vi "Set Object Size.vi"(4 "Set Width?":bool=TRUE, 6 "Set Height?":bool=TRUE, 7 "Cluster Border Correction":i32, 8 "error in (no error)":errorcluster, 9 "Size":cluster{"width":i16, "height":i16}, 10 "Size":i16, 11 "GObj Refnum":refnum<vi>) -> (0 "error out":errorcluster)   [LabVIEW 2021, in "IObject.lvclass"]
uses:
  IObject.lvclass
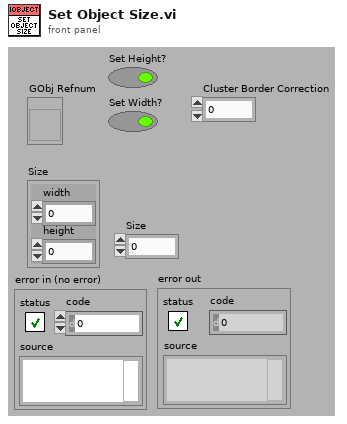
[diagram p1: front panel]
types:
  T1 = typedef "LVBoundsTypeDef.ctl" = cluster{"Width":u32, "Height":u32}
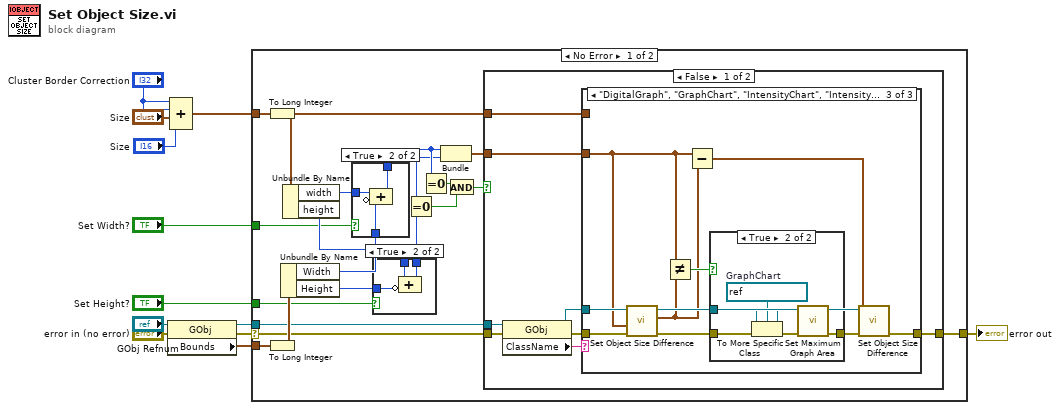
[diagram p0: block diagram]
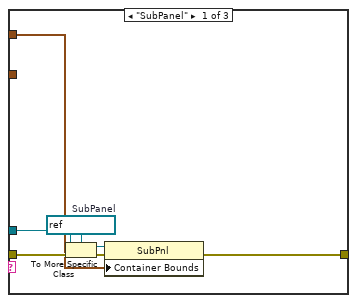
[diagram p2: hidden frame]
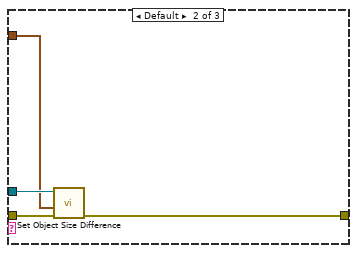
[diagram p3: hidden frame]
diagram:
  n1 = property class="GObj"(reference="GObj Refnum", error in="error in (no error)") -> (reference out=w1:refnum<vi>, error out=w2:errorcluster, "Bounds"=w10:T1)
  n2 = Compound Arithmetic op=unknown("Cluster Border Correction", "Cluster Border Correction", "Size", "Size") -> (w7:cluster{"width":i32, "height":i32})
  n3 = case shown="No Error" w2 {
    selector: w2 -> [w19 w74]
    tunnel: w7 -> [w17 _]
    tunnel: [w26 w74] -> w12
    tunnel: w10 -> [w30 _]
    tunnel: "Set Width?" -> [w22 _]
    tunnel: "Set Height?" -> [w21 _]
    tunnel: w1 -> [w18 _]
    frame No Error {
      n4 = To Long Integer(number=w17) -> (32bit integer=w16:cluster{"width":i32, "height":i32})
      n5 = To Long Integer(number=w30) -> (32bit integer=w31:cluster{"Width":i32, "Height":i32})
      n6 = Unbundle By Name(w31) -> ("Width"=w29:i32, "Height"=w25:i32)
      n7 = Unbundle By Name(w16) -> ("width"=w28:i32, "height"=w27:i32)
      n8 = case shown="True" w22 {
        tunnel: [_ w70] -> w15
        tunnel: w29 -> [_ w69]
        tunnel: w28 -> [_ w68]
        frame False {
        }
        frame True {
          n9 = Compound Arithmetic op=ADD(w68, invert w69) -> (w70:i32)
        }
      }
      n10 = case shown="True" w21 {
        tunnel: [_ w73] -> w14
        tunnel: w27 -> [_ w72]
        tunnel: w25 -> [_ w71]
        frame False {
        }
        frame True {
          n11 = Compound Arithmetic op=ADD(w72, invert w71) -> (w73:i32)
        }
      }
      n12 = Equal To 0?(x=w14) -> (x = 0?=w23:bool)
      n13 = Equal To 0?(x=w15) -> (x = 0?=w24:bool)
      n14 = Bundle(w15, w14) -> (w13:cluster{i32, i32})  [unwired: 1 in]
      n15 = And(x=w24, y=w23) -> (x .and. y?=w20:bool)
      n16 = case shown="False" w20 {
        tunnel: [w39 w67] -> w26
        tunnel: w19 -> [w38 w67]
        tunnel: w18 -> [w36 _]
        tunnel: w16 -> [w33 _]
        tunnel: w13 -> [w32 _]
        frame False {
          n17 = property class="GObj"(reference=w36, error in=w38) -> (reference out=w34:refnum<vi>, error out=w37:errorcluster, "ClassName"=w35:string)
          n18 = case shown="\"DigitalGraph\", \"GraphChart\", \"IntensityChart\", \"IntensityGraph\", \"MixedSignalGraph\", \"WaveformChart\", \"WaveformGraph\", \"XYGraph\"" w35 {
            tunnel: [w45 w48 w56] -> w39
            tunnel: w37 -> [w46 w49 w59]
            tunnel: w34 -> [w44 w50 w54]
            tunnel: w33 -> [w40 _ _]
            tunnel: w32 -> [_ w47 w53]
            frame "SubPanel" {
              w43 = refnum<vi> refnum  # SubPanel
              n19 = To More Specific Class(target class=w43, reference=w44, error in=w46) -> (specific class reference=w41:refnum<vi>, error out=w42:errorcluster)
              n20 = property class="SubPnl"(reference=w41, error in=w42, "Container Bounds"=w40) -> (error out=w45:errorcluster)  [unwired: 1 out]
            }
            frame Default {
              n21 = call "Set Object Size Difference.vi"("error in (no error)"=w49, "dSize"=w47, "GObj Refnum"=w50) -> ("error out"=w48:errorcluster)  [unwired: 7 in, 1 out]
            }
            frame "DigitalGraph", "GraphChart", "IntensityChart", "IntensityGraph", "MixedSignalGraph", "WaveformChart", "WaveformGraph", "XYGraph" {
              n22 = call "Set Object Size Difference.vi"("error in (no error)"=w59, "dSize"=w53, "GObj Refnum"=w54) -> ("error out"=w58:errorcluster, "dSize"=w52:cluster{"width":i32, "height":i32})  [unwired: 7 in]
              n23 = Not Equal?(x=w53, y=w52) -> (x != y?=w57:bool)
              n24 = Subtract(x=w53, y=w52) -> (x-y=w51:cluster{i32, i32})
              n25 = case shown="True" w57 {
                tunnel: [w60 w66] -> w55
                tunnel: w54 -> [_ w65]
                tunnel: w58 -> [w60 w63]
                frame False {
                }
                frame True {
                  w61 = refnum<vi> refnum  # GraphChart
                  n26 = To More Specific Class(target class=w61, reference=w65, error in=w63) -> (specific class reference=w64:refnum<vi>, error out=w62:errorcluster)
                  n27 = call "Set Maximum Graph Area.vi"("error in (no error)"=w62, "Waveform Chart"=w64) -> ("error out"=w66:errorcluster)  [unwired: 9 in]
                }
              }
              n28 = call "Set Object Size Difference.vi"("error in (no error)"=w55, "dSize"=w51, "GObj Refnum"=w54) -> ("error out"=w56:errorcluster)  [unwired: 7 in, 1 out]
            }
          }
        }
        frame True {
        }
      }
    }
    frame Error {
    }
  }
  "error out" <- w12
